vi "TestDoSampleCalibration.vi"() -> ()   [LabVIEW 2019]
uses:
  enable_disable_enum_typedef.ctl
  MotorController.lvclass
panel:
  out "Error Out":errorcluster
  in  "Serial Port":refnum<visa-resource-name>
  in  "Error In":errorcluster
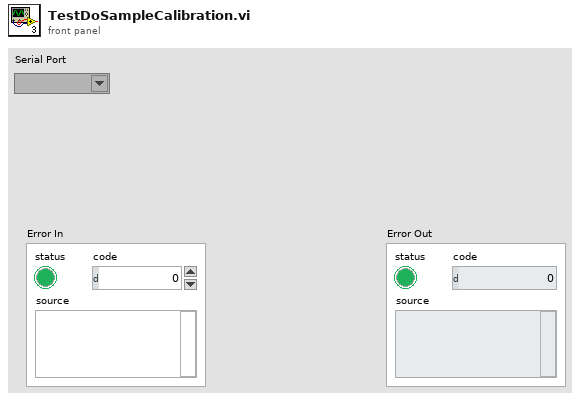
[diagram p1: front panel]
types:
  T1 = typedef "MotorController.lvclass/enable_disable_enum_typedef.ctl" = enum16{"Enable", "Disable"}
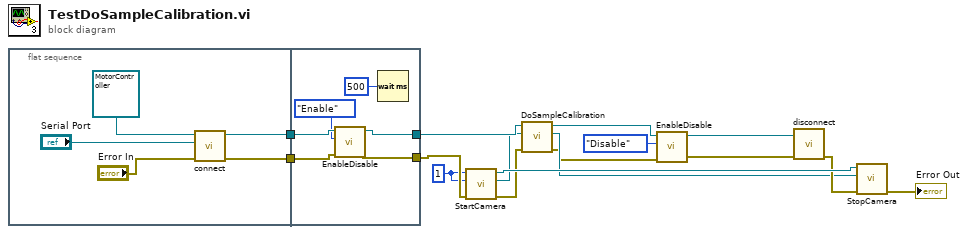
[diagram p0: block diagram]
diagram:
  w13 = u32 1 ("Gain")
  n1 = flat-sequence {
    tunnel: [w19] -> w16
    tunnel: [w18] -> w15
    tunnel: [w26] -> w6
    tunnel: w16 -> [w24]
    tunnel: w15 -> [w23]
    tunnel: [w25] -> w14
    frame #0 {
      n2 = call "connect.vi"("error in (no error)"="Error In", "Serial Port"="Serial Port", "MotorController in"=refnum<class "MotorController.lvclass"> refnum ("MotorController.lvclass")) -> ("error out"=w18:errorcluster, "MotorController out"=w19:refnum<class "MotorController.lvclass">)  [unwired: 7 in]
    }
    frame #1 {
      n3 = call "EnableDisable.vi"("error in (no error)"=w23, "Action"=enable_disable_enum_typedef."Enable", "MotorController in"=w24) -> ("error out"=w25:errorcluster, "MotorController out"=w26:refnum<class "MotorController.lvclass">)  [unwired: 7 in]
      n4 = Wait (ms)(milliseconds to wait=u32 500) -> ()  [unwired: 1 out]
    }
  }
  n5 = call "StartCamera.vi"("Error In"=w14, "ExposureTime_us"=w13, "Gain"=w13) -> ("Error Out"=w1:errorcluster, "TLCamera reference out"=w5:refnum<k24>, "TLCameraSDK reference out"=w12:refnum<k24>)  [unwired: 6 in]
  n6 = call "DoSampleCalibration.vi"("Error In"=w1, "TLCamera reference in"=w5, "MotorController in"=w6) -> ("Error Out"=w2:errorcluster, "TLCamera reference out"=w4:refnum<k24>, "MotorController out"=w3:refnum<class "MotorController.lvclass">)  [unwired: 6 in]
  n7 = call "EnableDisable.vi"("error in (no error)"=w2, "Action"=enable_disable_enum_typedef."Disable", "MotorController in"=w3) -> ("error out"=w8:errorcluster, "MotorController out"=w9:refnum<class "MotorController.lvclass">)  [unwired: 7 in]
  n8 = call "disconnect.vi"("error in (no error)"=w8, "MotorController in"=w9) -> ("error out"=w11:errorcluster)  [unwired: 8 in, 1 out]
  n9 = call "StopCamera.vi"("Error In"=w11, "TLCamera reference"=w4, "TLCameraSDK reference"=w12) -> ("Error Out"=→"Error Out":errorcluster)  [unwired: 8 in]
